vi "Application Paths.vi"(0 "FlexWorktable in":refnum<class "FlexWorktable.lvclass">, 1 "Project Path in":path, 5 "error in (no error)":errorcluster, 6 "Get/Set":enum16{"Get", "Set"}(ring)) -> (13 "Data Path":path, 14 "FlexWorktable out":refnum<class "FlexWorktable.lvclass">, 15 "Project Path":path, 16 "Config Path":path, 17 "Logs Path":path, 18 "Scripts Path":path, 19 "error out":errorcluster)   [LabVIEW 2023, in "FlexWorktable.lvclass"]
uses:
  FlexWorktable.lvclass
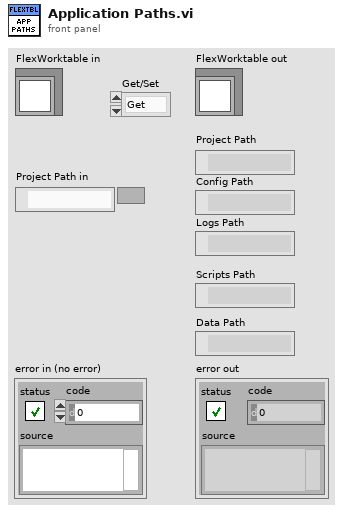
[diagram p1: front panel]
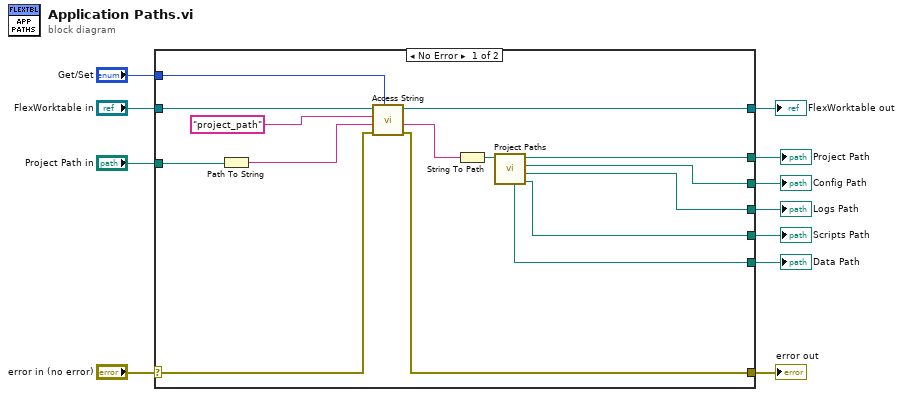
[diagram p0: block diagram]
diagram:
  n1 = case shown="No Error" "error in (no error)" {
    selector: "error in (no error)" -> [w25 w28]
    tunnel: [w18 w28] -> w10
    tunnel: [w16 w27] -> w8
    tunnel: "FlexWorktable in" -> [w26 w27]
    tunnel: "Project Path in" -> [w22 _]
    tunnel: "Get/Set" -> [w23 _]
    tunnel: [w17 _] -> w5
    tunnel: [w15 _] -> w4
    tunnel: [w14 _] -> w3
    tunnel: [w13 _] -> w2
    tunnel: [w12 _] -> w1
    frame No Error {
      n2 = Path To String(path=w22) -> (string=w21:string)
      n3 = call-dynamic "Access String.vi"("Get/Set"=w23, "error in (no error)"=w25, "Value in"=w21, "Key"="project_path", "FlexWorktable in"=w26) -> ("error out"=w18:errorcluster, "Value out"=w20:string, "FlexWorktable out"=w16:refnum<class "FlexWorktable.lvclass">)  [unwired: 4 in]
      n4 = String To Path(string=w20) -> (path=w19:path)
      n5 = call "Project Paths.vi"("Project Path in"=w19) -> ("Scripts Path"=w13:path, "Logs Path"=w14:path, "Config Path"=w15:path, "Project Path"=w17:path, "Data Path"=w12:path)  [unwired: 6 in]
    }
    frame Error {
    }
  }
  "error out" <- w10
  "FlexWorktable out" <- w8
  "Project Path" <- w5
  "Config Path" <- w4
  "Logs Path" <- w3
  "Scripts Path" <- w2
  "Data Path" <- w1
